vi "OldInterfaceGlue.vi"(8 "error in (no error)":errorcluster, 11 "ParsedData":T7) -> (0 "error out":errorcluster, 1 "IDs":T1, 2 "Parsing Data":T6, 3 "Image Size":cluster{"Width":dbl, "Height":dbl})   [LabVIEW 2019]
uses:
  ParseVectorFile/Typedefs/PublicEvents--ParseVectorFile.ParsedData.ctl
  Image/SVGImage.lvclass
  ParsePaths/Path.lvclass
  Rectangle/Rectangle.lvclass
  Dot/Dot.lvclass
  subVIs/typedefs/Parsed Path - Cluster.ctl
  <vilib>/Analysis/Matrix/Datatypes/RealMatrix.ctl
  subVIs/typedefs/Parsed Funnel - Cluster.ctl
  subVIs/typedefs/Parsed Rect - Cluster.ctl
  Image/SVGImage.lvclass/SVGImage.ctl
  Rectangle/Rectangle.lvclass/Rectangle.ctl
  Transform/Transform.lvclass/Transform.ctl
  ParsePaths/Path.lvclass/Path.ctl
  <vilib>/Analysis/baseanly.llb/Real A x B.vi
  Rectangle/Read Style.vi
  Rectangle/Read Width.vi
  Rectangle/Read Height.vi
  Rectangle/Read X.vi
  Rectangle/Read Y.vi
  Rectangle/Read Transforms.vi
  ParsePaths/Read Style.vi
  ParsePaths/Read Path Commands.vi
  ParsePaths/Read Transforms.vi
  Image/Read Width.vi
  Image/Read Height.vi
  <vilib>/Analysis/Matrix/Comparison/Not Equal/Not Equal - RM,RM.vi
  CSSProperties/CSSProperties.lvclass
  Transform/Transform.lvclass
  PathCommands/PathCommands.lvclass
  <vilib>/Analysis/Matrix/NI_Matrix.lvlib
  <vilib>/Analysis/NI_AALBase.lvlib
  ParseVectorFile/ParseVectorFile.lvclass
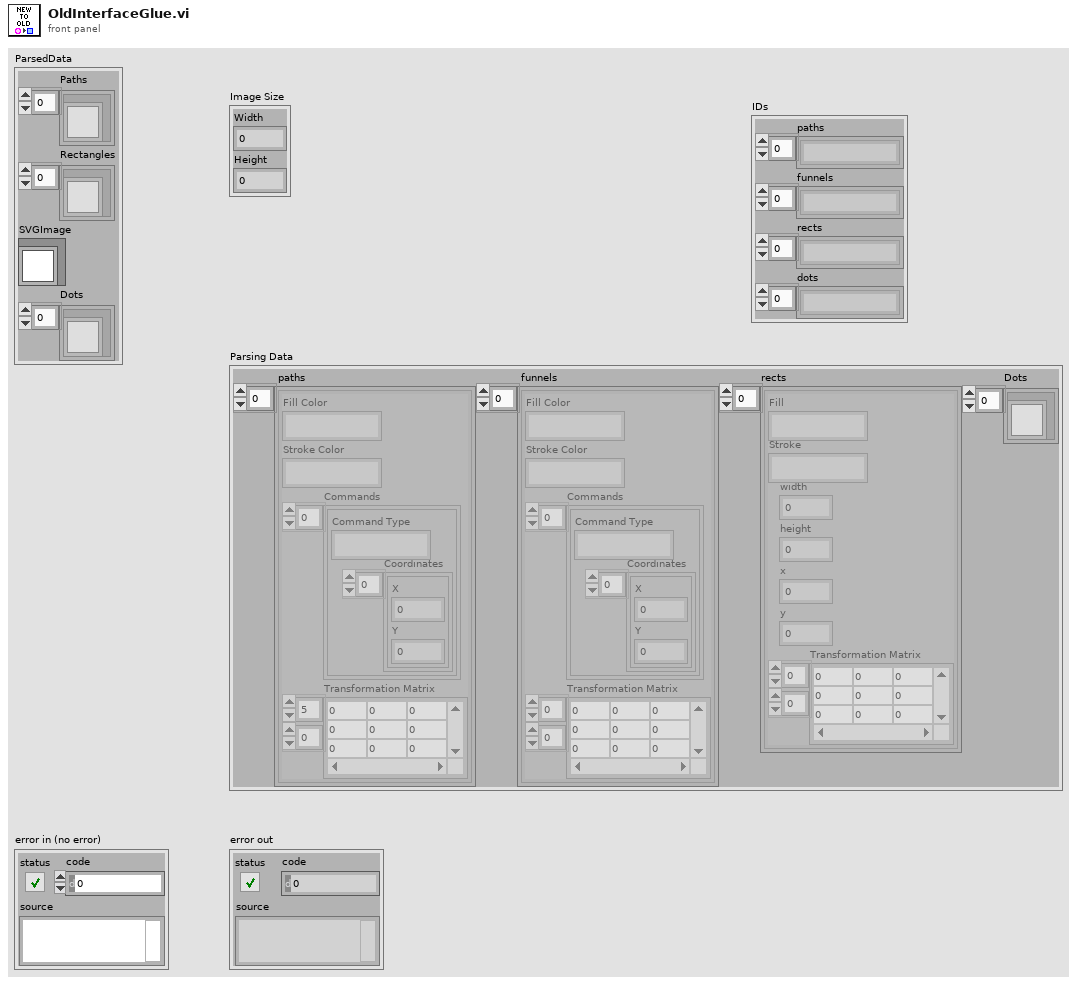
[diagram p1: front panel]
types:
  T1 = cluster{"paths":string[], "funnels":string[], "rects":string[], "dots":string[]}
  T2 = typedef "Parsed Path - Cluster.ctl" = cluster{"Fill Color":string, "Stroke Color":string, "Commands":cluster{"Command Type":string, "Coordinates":cluster{"X":dbl, "Y":dbl}[]}[], "Transformation Matrix":T3}
  T3 = typedef "NI_Matrix.lvlib/RealMatrix.ctl" = dbl[][]
  T4 = typedef "Parsed Funnel - Cluster.ctl" = cluster{"Fill Color":string, "Stroke Color":string, "Commands":cluster{"Command Type":string, "Coordinates":cluster{"X":dbl, "Y":dbl}[]}[], "Transformation Matrix":T3}
  T5 = typedef "Parsed Rect - Cluster.ctl" = cluster{"Fill":string, "Stroke":string, "width":dbl, "height":dbl, "x":dbl, "y":dbl, "Transformation Matrix":T3}
  T6 = cluster{" paths":T2[], " funnels":T4[], "rects":T5[], "Dots":refnum<class "Dot.lvclass">[]}
  T7 = typedef "ParseVectorFile.lvclass/PublicEvents--ParseVectorFile.ParsedData.ctl" = cluster{"Paths":refnum<class "Path.lvclass">[], "Rectangles":refnum<class "Rectangle.lvclass">[], "SVGImage":refnum<class "SVGImage.lvclass">, "Dots":refnum<class "Dot.lvclass">[]}
  T8 = cluster{"Fill":string, "Stroke":string, "Commands":cluster{"Command Type":string, "Coordinates":cluster{"X":dbl, "Y":dbl}[]}[], "Transformation Matrix":T3}
  T9 = cluster{"Command Type":string, "Coordinates":cluster{"X":dbl, "Y":dbl}[]}
  T10 = typedef "PathCommands.lvclass/Point.ctl" = cluster{"X":dbl, "Y":dbl}
  T11 = cluster{"Fill":string, "Stroke":string, "width":dbl, "height":dbl, "x":dbl, "y":dbl, "Transformation Matrix":T3}
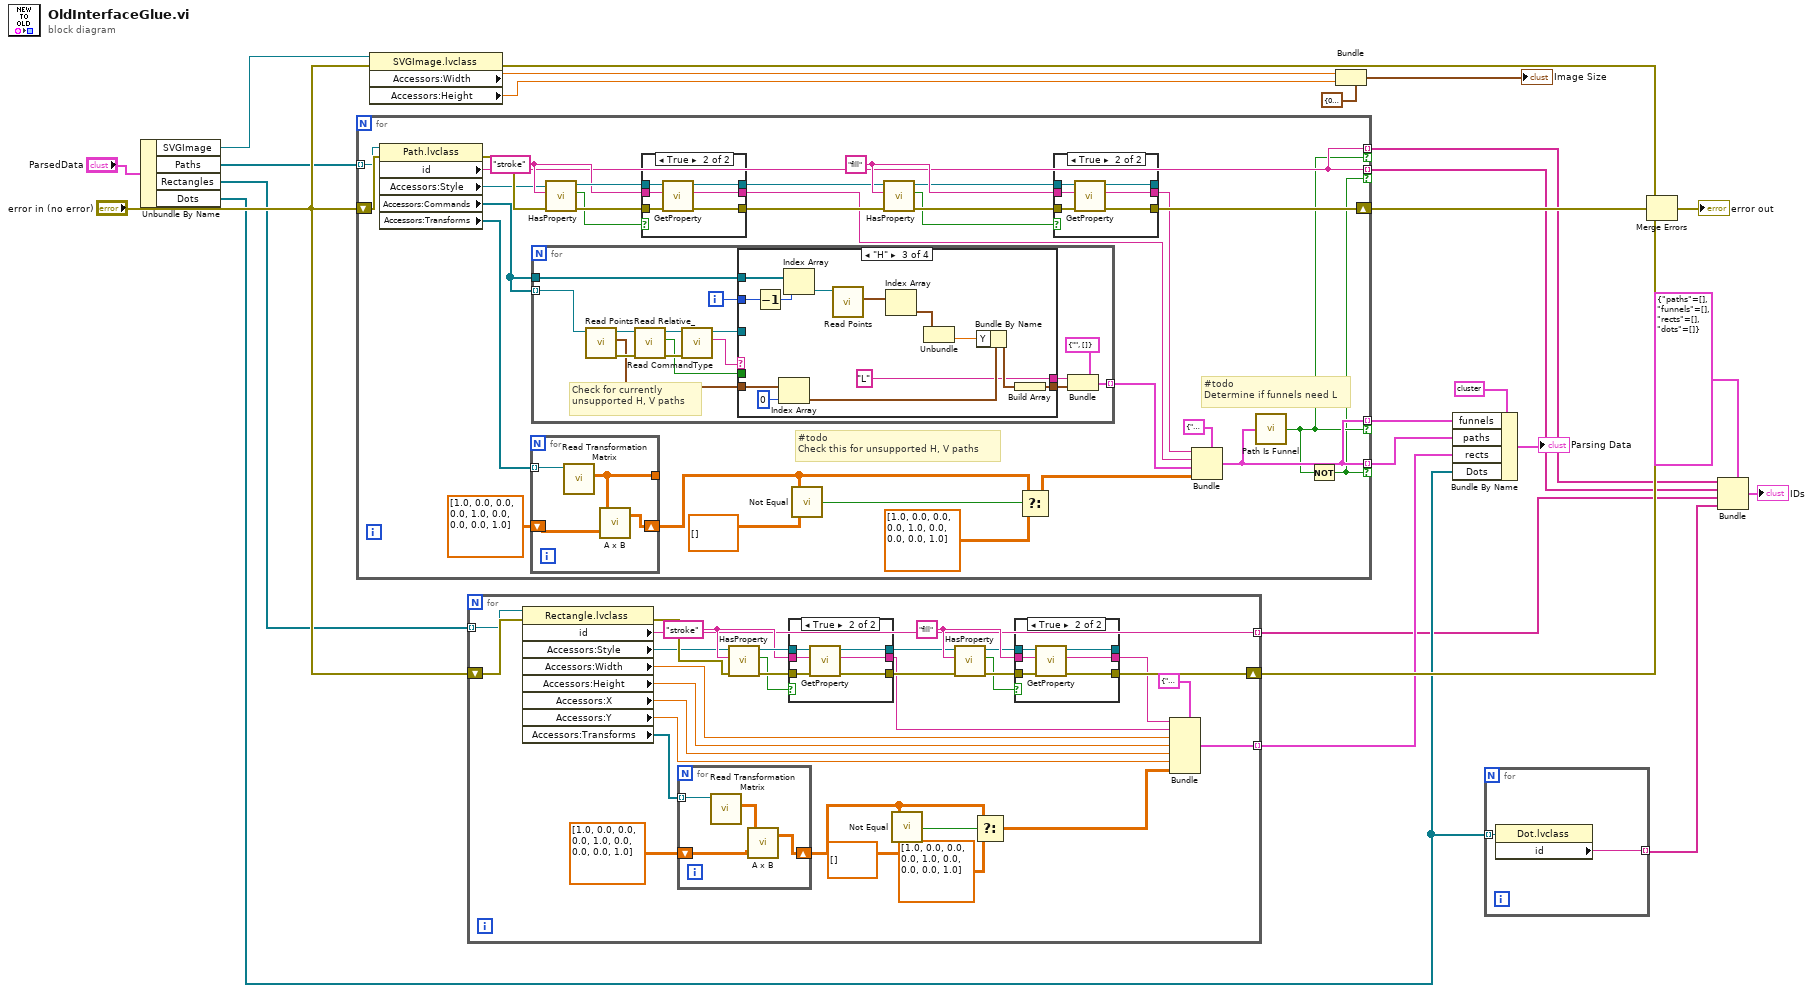
[diagram p0: block diagram]
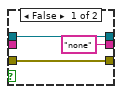
[diagram p2: hidden frame]
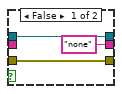
[diagram p3: hidden frame]
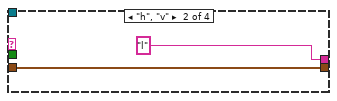
[diagram p5: hidden frame]
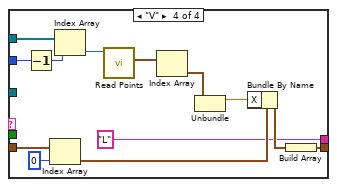
[diagram p6: hidden frame]
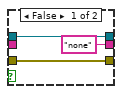
[diagram p7: hidden frame]
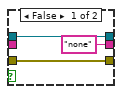
[diagram p8: hidden frame]
diagram:
  n1 = Unbundle By Name("ParsedData") -> ("SVGImage"=w17:refnum<class "SVGImage.lvclass">, "Paths"=w19:refnum<class "Path.lvclass">[], "Rectangles"=w18:refnum<class "Rectangle.lvclass">[], "Dots"=w7:refnum<class "Dot.lvclass">[])
  n2 = for {
    tunnel: w19 -> [w41] mode=indexing
    tunnel: [w42] -> w10 mode=indexing if=w27
    tunnel: [w42] -> w11 mode=indexing if=w26
    shift-right: [w52] -> w24
    shift-left: "error in (no error)" -> [w53]
    tunnel: [w28] -> w6 mode=indexing if=w27
    tunnel: [w28] -> w5 mode=indexing if=w26
    w46 = "fill" ("Property")
    w49 = "stroke" ("Property")
    # "#todo\nDetermine if funnels need L"
    # "#todo\nCheck this for unsupported H, V paths"
    n3 = property class="Path.lvclass"(reference=w41, error in=w53) -> (error out=w51:errorcluster, "id"=w28:string, "Accessors:Style"=w40:refnum<class "CSSProperties.lvclass">, "Accessors:Commands"=w35:refnum<class "PathCommands.lvclass">[], "Accessors:Transforms"=w39:refnum<class "Transform.lvclass">[])  [unwired: 1 out]
    n4 = for {
      tunnel: w39 -> [w60] mode=indexing
      tunnel: [w59] -> _
      shift-right: [w57] -> w29
      shift-left: T3 [[1.0, 0.0, 0.0], [0.0, 1.0, 0.0], [0.0, 0.0, 1.0]] ("Real Matrix") -> [w58]
      n5 = call "Read Transformation Matrix.vi"("Transform in"=w60) -> ("Real Matrix"=w59:T3)  [unwired: 8 in, 2 out]
      n6 = call-poly <vilib>:"A x B.vi"("B"=w58, "A"=w59) -> ("A x B"=w57:T3)  [unwired: 1 out]
    }
    n7 = for {
      tunnel: w35 -> [w71] mode=indexing
      tunnel: [w75] -> w38 mode=indexing
      tunnel: w35 -> [w67]
      i -> [w65]
      # "Check for currently unsupported H, V paths"
      n8 = call-dynamic "Read Points.vi"("PathCommands in"=w71) -> ("error out"=w70:errorcluster, "Points"=w64:T10[], "PathCommands out"=w73:refnum<class "PathCommands.lvclass">)  [unwired: 8 in]
      n9 = call-dynamic "Read Relative_.vi"("error in (no error)"=w70, "PathCommands in"=w73) -> ("error out"=w69:errorcluster, "Relative?"=w63:bool, "PathCommands out"=w72:refnum<class "PathCommands.lvclass">)  [unwired: 7 in]
      n10 = call-dynamic "Read CommandType.vi"("error in (no error)"=w69, "PathCommands in"=w72) -> ("CommandType"=w66:string, "PathCommands out"=w68:refnum<class "PathCommands.lvclass">)  [unwired: 7 in, 1 out]
      n11 = case shown="\"H\"" w66 {
        selector: w66 -> [w77 _ _ _]
        tunnel: w68 -> [_ _ _ _]
        tunnel: w67 -> [_ _ w92 w105]
        tunnel: w65 -> [_ _ w91 w104]
        tunnel: w64 -> [w76 w79 w87 w100]
        tunnel: w63 -> [_ _ _ _]
        tunnel: [w76 w79 w82 w95] -> w62
        tunnel: [w77 "l" "L" "L"] -> w61
        frame Default {
        }
        frame "h", "v" {
        }
        frame "H" {
          n12 = Decrement(x=w91) -> (x-1=w90:i32)
          n13 = Index Array(array=w87, index=0) -> (element=w84:T10)
          n14 = Index Array(array=w92, index=w90) -> (element=w89:refnum<class "PathCommands.lvclass">)
          n15 = call-dynamic "Read Points.vi"("PathCommands in"=w89) -> ("Points"=w88:T10[])  [unwired: 8 in, 2 out]
          n16 = Index Array(array=w88) -> (element=w85:T10)  [unwired: 1 in]
          n17 = Unbundle(w85) -> ("Y"=w80:dbl)  [unwired: 1 out]
          n18 = Bundle By Name(cluster=w84, "Y"=w80) -> (w83:T10)
          n19 = Build Array(w83) -> (w82:T10[])
        }
        frame "V" {
          n20 = Decrement(x=w104) -> (x-1=w103:i32)
          n21 = Index Array(array=w100, index=0) -> (element=w97:T10)
          n22 = Index Array(array=w105, index=w103) -> (element=w102:refnum<class "PathCommands.lvclass">)
          n23 = call-dynamic "Read Points.vi"("PathCommands in"=w102) -> ("Points"=w101:T10[])  [unwired: 8 in, 2 out]
          n24 = Index Array(array=w101) -> (element=w98:T10)  [unwired: 1 in]
          n25 = Unbundle(w98) -> ("X"=w93:dbl)  [unwired: 1 out]
          n26 = Bundle By Name(cluster=w97, "X"=w93) -> (w96:T10)
          n27 = Build Array(w96) -> (w95:T10[])
        }
      }
      n28 = Bundle(cluster=T9 {"Command Type"="", "Coordinates"=[]} ("Command"), "Command Type"=w61, "Coordinates"=w62) -> (w75:T9)
    }
    n29 = call "HasProperty.vi"("error in (no error)"=w51, "Property"=w49, "CSSProperties in"=w40) -> ("error out"=w56:errorcluster, "Exists?"=w48:bool, "CSSProperties out"=w50:refnum<class "CSSProperties.lvclass">)  [unwired: 6 in]
    n30 = case shown="True" w48 {
      tunnel: [w116 w121] -> w44
      tunnel: ["none" ("Value") w120] -> w36
      tunnel: w50 -> [w116 w119]
      tunnel: w49 -> [_ w118]
      tunnel: w56 -> [w117 w123]
      tunnel: [w117 w122] -> w54
      frame False {
      }
      frame True {
        n31 = call "GetProperty.vi"("error in (no error)"=w123, "Property"=w118, "CSSProperties in"=w119) -> ("error out"=w122:errorcluster, "Value"=w120:string, "CSSProperties out"=w121:refnum<class "CSSProperties.lvclass">)  [unwired: 6 in]
      }
    }
    n32 = call-poly <vilib>:"Not Equal.vi"("Real Matrix B"=T3 [] ("Real Matrix"), "Real Matrix A"=w29) -> ("A != B?"=w34:bool)
    n33 = call "HasProperty.vi"("error in (no error)"=w54, "Property"=w46, "CSSProperties in"=w44) -> ("error out"=w55:errorcluster, "Exists?"=w47:bool, "CSSProperties out"=w45:refnum<class "CSSProperties.lvclass">)  [unwired: 6 in]
    n34 = Select(t=w29, s=w34, f=T3 [[1.0, 0.0, 0.0], [0.0, 1.0, 0.0], [0.0, 0.0, 1.0]] ("Real Matrix")) -> (s? t:f=w32:T3)
    n35 = case shown="True" w47 {
      tunnel: [w107 w112] -> _
      tunnel: ["none" ("Value") w111] -> w37
      tunnel: w45 -> [w107 w110]
      tunnel: w46 -> [_ w109]
      tunnel: w55 -> [w108 w114]
      tunnel: [w108 w113] -> w52
      frame False {
      }
      frame True {
        n36 = call "GetProperty.vi"("error in (no error)"=w114, "Property"=w109, "CSSProperties in"=w110) -> ("error out"=w113:errorcluster, "Value"=w111:string, "CSSProperties out"=w112:refnum<class "CSSProperties.lvclass">)  [unwired: 6 in]
      }
    }
    n37 = Bundle(cluster=T8 {"Fill"="", "Stroke"="", "Commands"=[], "Transformation Matrix"=[]} ("Path Information"), "Fill"=w37, "Stroke"=w36, "Commands"=w38, "Transformation Matrix"=w32) -> (w42:T8)
    n38 = call "Path Is Funnel.vi"("Path Information"=w42) -> ("Is Funnel?"=w27:bool)
    n39 = Not(x=w27) -> (.not. x?=w26:bool)
  }
  n40 = property class="SVGImage.lvclass"(reference=w17, error in="error in (no error)") -> (error out=w22:errorcluster, "Accessors:Width"=w15:dbl, "Accessors:Height"=w14:dbl)  [unwired: 1 out]
  n41 = for {
    tunnel: w18 -> [w148] mode=indexing
    tunnel: [w139] -> w9 mode=indexing
    shift-right: [w149] -> w21
    shift-left: "error in (no error)" -> [w151]
    tunnel: [w124] -> w4 mode=indexing
    w143 = "fill" ("Property")
    w146 = "stroke" ("Property")
    n42 = property class="Rectangle.lvclass"(reference=w148, error in=w151) -> (error out=w150:errorcluster, "id"=w124:string, "Accessors:Style"=w140:refnum<class "CSSProperties.lvclass">, "Accessors:Width"=w134:dbl, "Accessors:Height"=w135:dbl, "Accessors:X"=w136:dbl, "Accessors:Y"=w137:dbl, "Accessors:Transforms"=w138:refnum<class "Transform.lvclass">[])  [unwired: 1 out]
    n43 = for {
      tunnel: w138 -> [w158] mode=indexing
      shift-right: [w155] -> w125
      shift-left: T3 [[1.0, 0.0, 0.0], [0.0, 1.0, 0.0], [0.0, 0.0, 1.0]] ("Real Matrix") -> [w157]
      n44 = call "Read Transformation Matrix.vi"("Transform in"=w158) -> ("Real Matrix"=w156:T3)  [unwired: 8 in, 2 out]
      n45 = call-poly <vilib>:"A x B.vi"("B"=w157, "A"=w156) -> ("A x B"=w155:T3)  [unwired: 1 out]
    }
    n46 = call "HasProperty.vi"("error in (no error)"=w150, "Property"=w146, "CSSProperties in"=w140) -> ("error out"=w154:errorcluster, "Exists?"=w145:bool, "CSSProperties out"=w147:refnum<class "CSSProperties.lvclass">)  [unwired: 6 in]
    n47 = case shown="True" w145 {
      tunnel: [w169 w174] -> w141
      tunnel: ["none" ("Value") w173] -> w132
      tunnel: w147 -> [w169 w172]
      tunnel: w146 -> [_ w171]
      tunnel: w154 -> [w170 w176]
      tunnel: [w170 w175] -> w152
      frame False {
      }
      frame True {
        n48 = call "GetProperty.vi"("error in (no error)"=w176, "Property"=w171, "CSSProperties in"=w172) -> ("error out"=w175:errorcluster, "Value"=w173:string, "CSSProperties out"=w174:refnum<class "CSSProperties.lvclass">)  [unwired: 6 in]
      }
    }
    n49 = call-poly <vilib>:"Not Equal.vi"("Real Matrix B"=T3 [] ("Real Matrix"), "Real Matrix A"=w125) -> ("A != B?"=w130:bool)
    n50 = call "HasProperty.vi"("error in (no error)"=w152, "Property"=w143, "CSSProperties in"=w141) -> ("error out"=w153:errorcluster, "Exists?"=w144:bool, "CSSProperties out"=w142:refnum<class "CSSProperties.lvclass">)  [unwired: 6 in]
    n51 = Select(t=w125, s=w130, f=T3 [[1.0, 0.0, 0.0], [0.0, 1.0, 0.0], [0.0, 0.0, 1.0]] ("Real Matrix")) -> (s? t:f=w128:T3)
    n52 = case shown="True" w144 {
      tunnel: [w160 w165] -> _
      tunnel: ["none" ("Value") w164] -> w133
      tunnel: w142 -> [w160 w163]
      tunnel: w143 -> [_ w162]
      tunnel: w153 -> [w161 w167]
      tunnel: [w161 w166] -> w149
      frame False {
      }
      frame True {
        n53 = call "GetProperty.vi"("error in (no error)"=w167, "Property"=w162, "CSSProperties in"=w163) -> ("error out"=w166:errorcluster, "Value"=w164:string, "CSSProperties out"=w165:refnum<class "CSSProperties.lvclass">)  [unwired: 6 in]
      }
    }
    n54 = Bundle(cluster=T11 {"Fill"="", "Stroke"="", "width"=12798.633, "height"=8237.7939, "x"=17571.604, "y"=12316.77, "Transformation Matrix"=[]}, "Fill"=w133, "Stroke"=w132, "width"=w134, "height"=w135, "x"=w136, "y"=w137, "Transformation Matrix"=w128) -> (w139:T11)
  }
  n55 = Bundle(cluster=cluster{"Width":dbl, "Height":dbl} {"Width"=0.0, "Height"=0.0} ("Image Size"), "Width"=w15, "Height"=w14) -> (→"Image Size":cluster{"Width":dbl, "Height":dbl})
  n56 = Bundle By Name(cluster=T6 {" paths"=[{"Fill Color"="none", "Stroke Color"="#00fb00", "Commands"=[{"Command Type"="M", "Coordinates"=[{"X"=11596.551, "Y"=15958.369}]}, {"Command Type"="C", "Coordinates"=[{"X"=11596.551, "Y"=15958.369}, {"X"=11590.232, "Y"=13296.496}, {"X"=11844.039, "Y"=11998.571}]}, {"Command Type"="C", "Coordinates"=[{"X"=12192.351, "Y"=10217.362}, {"X"=11976.551, "Y"=7839.6266}, {"X"=13576.45, "Y"=6836.692}]}, {"Command Type"="C", "Coordinates"=[{"X"=15287.894, "Y"=5763.8329}, {"X"=19886.993, "Y"=6255.5101}, {"X"=23051.681, "Y"=6129.5852}]}, {"Command Type"="C", "Coordinates"=[{"X"=25383.318, "Y"=6036.8079}, {"X"=27721.298, "Y"=5981.1511}, {"X"=30052.038, "Y"=6094.2299}]}, {"Command Type"="C", "Coordinates"=[{"X"=31554.801, "Y"=6167.1383}, {"X"=33380.219, "Y"=5598.0828}, {"X"=34542.166, "Y"=6553.8493}]}, {"Command Type"="C", "Coordinates"=[{"X"=35665.028, "Y"=7477.4665}, {"X"=35764.974, "Y"=9272.7169}, {"X"=35814.958, "Y"=10725.779}]}, {"Command Type"="C", "Coordinates"=[{"X"=35870.683, "Y"=12345.735}, {"X"=34718.943, "Y"=15463.395}, {"X"=34718.943, "Y"=15463.395}]}], "Transformation Matrix"=[]}], " funnels"=[{"Fill Color"="#00ff00", "Stroke Color"="#00fb00", "Commands"=[{"Command Type"="M", "Coordinates"=[{"X"=8892.9234, "Y"=16667.558}]}, {"Command Type"="L", "Coordinates"=[{"X"=8937.5164, "Y"=12073.802}]}, {"Command Type"="C", "Coordinates"=[{"X"=10398.541, "Y"=13045.785}, {"X"=11973.214, "Y"=13787.632}, {"X"=13619.827, "Y"=14383.805}]}, {"Command Type"="C", "Coordinates"=[{"X"=11867.015, "Y"=14727.874}, {"X"=10188.303, "Y"=15246.418}, {"X"=8892.9234, "Y"=16667.558}]}, {"Command Type"="z", "Coordinates"=[]}], "Transformation Matrix"=[]}, {"Fill Color"="#00ff00", "Stroke Color"="#00fb00", "Commands"=[{"Command Type"="M", "Coordinates"=[{"X"=17572.822, "Y"=3200.4476}]}, {"Command Type"="L", "Coordinates"=[{"X"=22166.578, "Y"=3245.0411}]}, {"Command Type"="C", "Coordinates"=[{"X"=21194.595, "Y"=4706.0654}, {"X"=20452.748, "Y"=6280.7391}, {"X"=19856.575, "Y"=7927.3519}]}, {"Command Type"="C", "Coordinates"=[{"X"=19512.506, "Y"=6174.5401}, {"X"=18993.962, "Y"=4495.8279}, {"X"=17572.822, "Y"=3200.4476}]}, {"Command Type"="z", "Coordinates"=[]}], "Transformation Matrix"=[]}, {"Fill Color"="#00ff00", "Stroke Color"="#00fb00", "Commands"=[{"Command Type"="M", "Coordinates"=[{"X"=24573.18, "Y"=3341.869}]}, {"Command Type"="L", "Coordinates"=[{"X"=29166.936, "Y"=3386.4625}]}, {"Command Type"="C", "Coordinates"=[{"X"=28194.953, "Y"=4847.4868}, {"X"=27453.106, "Y"=6422.1605}, {"X"=26856.933, "Y"=8068.7733}]}, {"Command Type"="C", "Coordinates"=[{"X"=26512.864, "Y"=6315.9615}, {"X"=25994.32, "Y"=4637.2493}, {"X"=24573.18, "Y"=3341.869}]}, {"Command Type"="z", "Coordinates"=[]}], "Transformation Matrix"=[]}, {"Fill Color"="#00ff00", "Stroke Color"="#00fb00", "Commands"=[{"Command Type"="M", "Coordinates"=[{"X"=8902.834, "Y"=9833.0681}]}, {"Command Type"="L", "Coordinates"=[{"X"=9838.4796, "Y"=5335.3853}]}, {"Command Type"="C", "Coordinates"=[{"X"=11082.987, "Y"=6572.5377}, {"X"=12483.662, "Y"=7605.9988}, {"X"=13983.191, "Y"=8510.5254}]}, {"Command Type"="C", "Coordinates"=[{"X"=12196.931, "Y"=8507.7297}, {"X"=10449.486, "Y"=8690.4757}, {"X"=8902.834, "Y"=9833.0681}]}, {"Command Type"="z", "Coordinates"=[]}], "Transformation Matrix"=[]}, {"Fill Color"="#00ff00", "Stroke Color"="#00fb00", "Commands"=[{"Command Type"="M", "Coordinates"=[{"X"=38224.873, "Y"=9271.1882}]}, {"Command Type"="L", "Coordinates"=[{"X"=37289.227, "Y"=4773.5052}]}, {"Command Type"="C", "Coordinates"=[{"X"=36044.72, "Y"=6010.6572}, {"X"=34644.045, "Y"=7044.1182}, {"X"=33144.516, "Y"=7948.6452}]}, {"Command Type"="C", "Coordinates"=[{"X"=34930.776, "Y"=7945.8492}, {"X"=36678.221, "Y"=8128.5952}, {"X"=38224.873, "Y"=9271.1882}]}, {"Command Type"="z", "Coordinates"=[]}], "Transformation Matrix"=[]}, {"Fill Color"="#00ff00", "Stroke Color"="#00fb00", "Commands"=[{"Command Type"="M", "Coordinates"=[{"X"=38072.344, "Y"=16204.638}]}, {"Command Type"="L", "Coordinates"=[{"X"=38027.751, "Y"=11610.882}]}, {"Command Type"="C", "Coordinates"=[{"X"=36566.727, "Y"=12582.865}, {"X"=34992.054, "Y"=13324.712}, {"X"=33345.441, "Y"=13920.885}]}, {"Command Type"="C", "Coordinates"=[{"X"=35098.253, "Y"=14264.954}, {"X"=36776.965, "Y"=14783.498}, {"X"=38072.344, "Y"=16204.638}]}, {"Command Type"="z", "Coordinates"=[]}], "Transformation Matrix"=[]}], "rects"=[{"Fill"="#00ff00", "Stroke"="#000000", "width"=12798.633, "height"=8237.7939, "x"=17571.604, "y"=12316.77, "Transformation Matrix"=[]}], "Dots"=[]} ("Parsing Data"), "funnels"=w10, "paths"=w11, "rects"=w9, "Dots"=w7) -> (→"Parsing Data":T6)
  n57 = for {
    tunnel: w7 -> [w178] mode=indexing
    tunnel: [w177] -> w3 mode=indexing
    n58 = property class="Dot.lvclass"(reference=w178) -> ("id"=w177:string)  [unwired: 1 in, 2 out]
  }
  n59 = Merge Errors(w22, w24, w21) -> (→"error out":errorcluster)
  n60 = Bundle(cluster=T1 {"paths"=[], "funnels"=[], "rects"=[], "dots"=[]}, "paths"=w6, "funnels"=w5, "rects"=w4, "dots"=w3) -> (→"IDs":T1)
